vi "K2182A_Set_Monitor_Values.vi"(5 "System Monitor Variables (in)":T1) -> (1 "System Monitor Variables (out)":T1)   [LabVIEW 2019]
uses:
  Global/Global Variables/System Monitor Cluster.ctl
  Global/Global Variables/Data_Display_global.vi
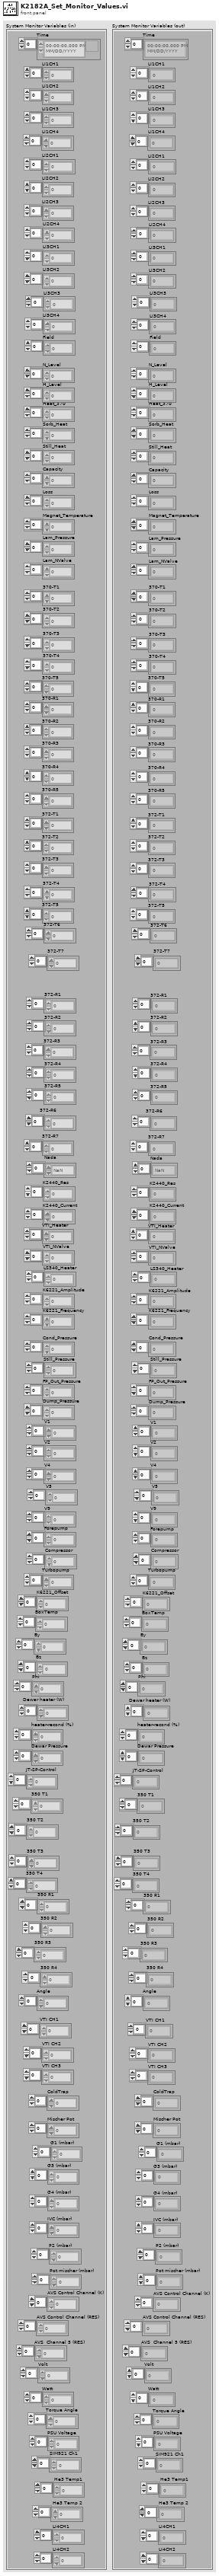
[diagram p1: front panel]
types:
  T1 = typedef "System Monitor Cluster.ctl" = cluster{"Time":timestamp[], "LI1CH1":dbl[], "LI1CH2":dbl[], "LI2CH1":dbl[], "LI2CH2":dbl[], "LI3CH1":dbl[], "LI3CH2":dbl[], "Field":dbl[], "N_Level":dbl[], "H_Level":dbl[], "Heat_370":dbl[], "Sorb_Heat":dbl[], "Still_Heat":dbl[], "Capacity":dbl[], "Loss":dbl[], "Magnet_Temperature":dbl[], "Lam_Pressure":dbl[], "Lam_NValve":dbl[], "370-T1":dbl[], "370-T2":dbl[], "370-T3":dbl[], "370-T4":dbl[], "370-T5":dbl[], "370-R1":dbl[], "370-R2":dbl[], "370-R3":dbl[], "370-R4":dbl[], "370-R5":dbl[], "372-T1":dbl[], "372-T2":dbl[], "372-T3":dbl[], "372-T4":dbl[], "372-T5":dbl[], "372-T6":dbl[], "372-R1":dbl[], "372-R2":dbl[], "372-R3":dbl[], "372-R4":dbl[], "372-R5":dbl[], "372-R6":dbl[], "Nada":dbl[], "K2440_Res":dbl[], "K2440_Current":dbl[], "VTI_Heater":dbl[], "VTI_NValve":dbl[], "LS340_Heater":dbl[], "K6221_Amplitude":dbl[], "K6221_Frequency":dbl[], "Cond_Pressure":dbl[], "Still_Pressure":dbl[], "FP_Out_Pressure":dbl[], "Dump_Pressure":dbl[], "V1":dbl[], "V2":dbl[], "V4":dbl[], "V5":dbl[], "V9":dbl[], "Forepump":dbl[], "Compressor":dbl[], "K6221_Offset":dbl[], "BoxTemp":dbl[], "By":dbl[], "Bz":dbl[], "Phi":dbl[], "heater-recond (%)":dbl[], "Dewar Pressure ":dbl[], "JT-SP-Control":dbl[], "350 T1":dbl[], "350 T2":dbl[], "350 T3":dbl[], "350 T4":dbl[], "350 R1":dbl[], "350 R2":dbl[], "350 R3":dbl[], "350 R4":dbl[], "Angle":dbl[], "VTI CH1":dbl[], "VTI CH2":dbl[], "VTI CH3":dbl[], "ColdTrap":dbl[], "Mischer Pot":dbl[], "G1 (mbar)":dbl[], "G3 (mbar) ":dbl[], "G4 (mbar)":dbl[], "IVC (mbar)":dbl[], "P2 (mbar) ":dbl[], "Pot mischer (mbar)":dbl[], "AVS Control Channel (K)":dbl[], "AVS Control Channel (RES)":dbl[], "AVS  Channel 5 (RES) ":dbl[], "LI3CH3":dbl[], "LI3CH4":dbl[], "LI1CH3":dbl[], "LI1CH4":dbl[], "LI2CH3":dbl[], "LI2CH4":dbl[], "Volt":dbl[], "Watt":dbl[], "Torque Angle":dbl[], "Dewar heater (W)":dbl[], "PSU Voltage":dbl[], "Turbopump":dbl[], "372-R7":dbl[], "372-T7":dbl[], "SIM921 Ch1":dbl[], " He3 Temp1":dbl[], " He3 Temp 2":dbl[], "LI4CH1":dbl[], "LI4CH2":dbl[]}
  T2 = typedef "K2812A_cluster.ctl" = cluster{"Plot Window":dbl[][], "Range":dbl, "Update":bool, "Range selector":T3, "Auto Range":bool, "V":dbl, "Auto Range set":bool}
  T3 = typedef "Keithley 622x.lvlib/KE2182 -- Voltage Ranges.ctl" = enum16{"10mV", "100mV", "1V", "10V", "100V"}
  T4 = typedef "K6221_Cluster.ctl" = cluster{"Plot Window":dbl[][], "A":dbl, "A (RMS)":dbl, "Hz":dbl, "I (A)":dbl, "f (Hz)":dbl, "Update":bool, "Offset":dbl, "Offset (A)":dbl, "Compliance":bool, "Output":bool, "Output Status":bool}
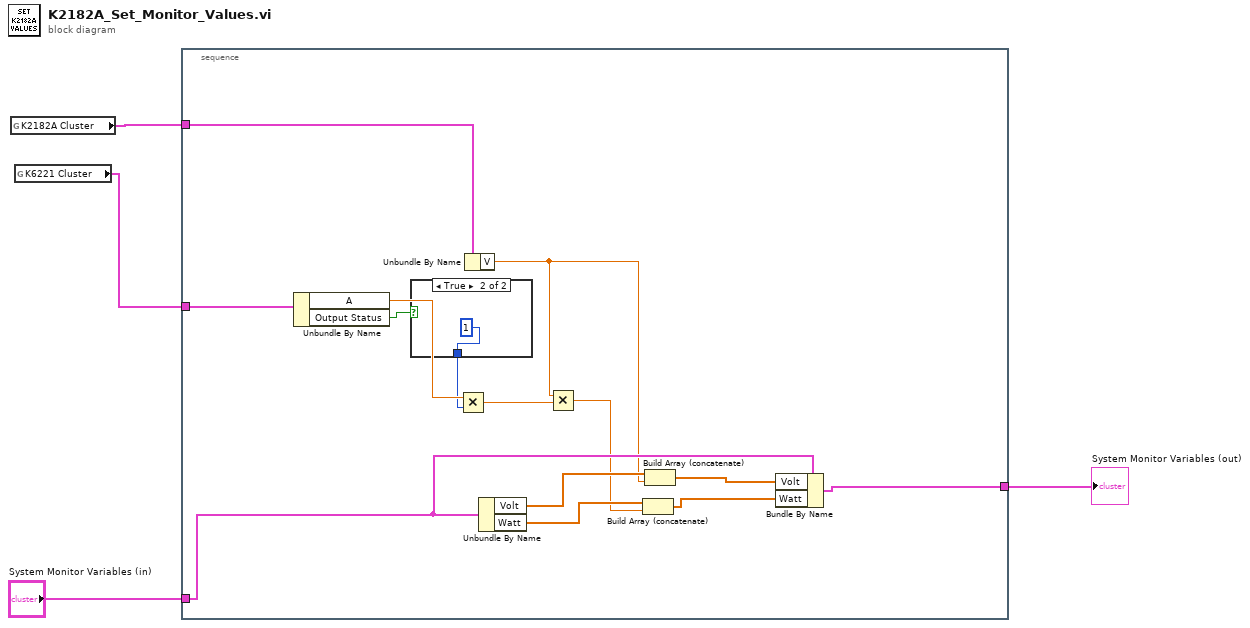
[diagram p0: block diagram]
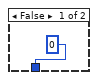
[diagram p2: hidden frame]
diagram:
  n1 = global read "Data_Display_global.vi" "K2182A Cluster"() -> (w3:T2)
  n2 = global read "Data_Display_global.vi" "K6221 Cluster"() -> (w1:T4)
  n3 = stacked-sequence {
    tunnel: "System Monitor Variables (in)" -> [w14]
    tunnel: w3 -> [w18]
    tunnel: [w16] -> w2
    tunnel: w1 -> [w11]
    frame #0 {
      n4 = Unbundle By Name(w11) -> ("A"=w7:dbl, "Output Status"=w8:bool)
      n5 = case shown="True" w8 {
        tunnel: [0 1] -> w5
        frame False {
        }
        frame True {
        }
      }
      n6 = Multiply(x=w7, y=w5) -> (x*y=w6:dbl)
      n7 = Unbundle By Name(w18) -> ("V"=w10:dbl)
      n8 = Unbundle By Name(w14) -> ("Volt"=w17:dbl[], "Watt"=w12:dbl[])
      n9 = Multiply(x=w10, y=w6) -> (x*y=w9:dbl)
      n10 = Build Array (concatenate)(w12, w9) -> (w13:dbl[])
      n11 = Build Array (concatenate)(w17, w10) -> (w15:dbl[])
      n12 = Bundle By Name(cluster=w14, "Volt"=w15, "Watt"=w13) -> (w16:T1)
    }
  }
  "System Monitor Variables (out)" <- w2
